vi "Get XY graph from TDMS file.vi"(8 "error in":errorcluster, 11 "TDMS file path":path) -> (0 "error out":errorcluster, 1 "graph":cluster{"X":dbl[], "Y":dbl[]}[](graph), 3 "TDMS file path out":path)   [LabVIEW 2025]
panel:
  out "Numeric":i32
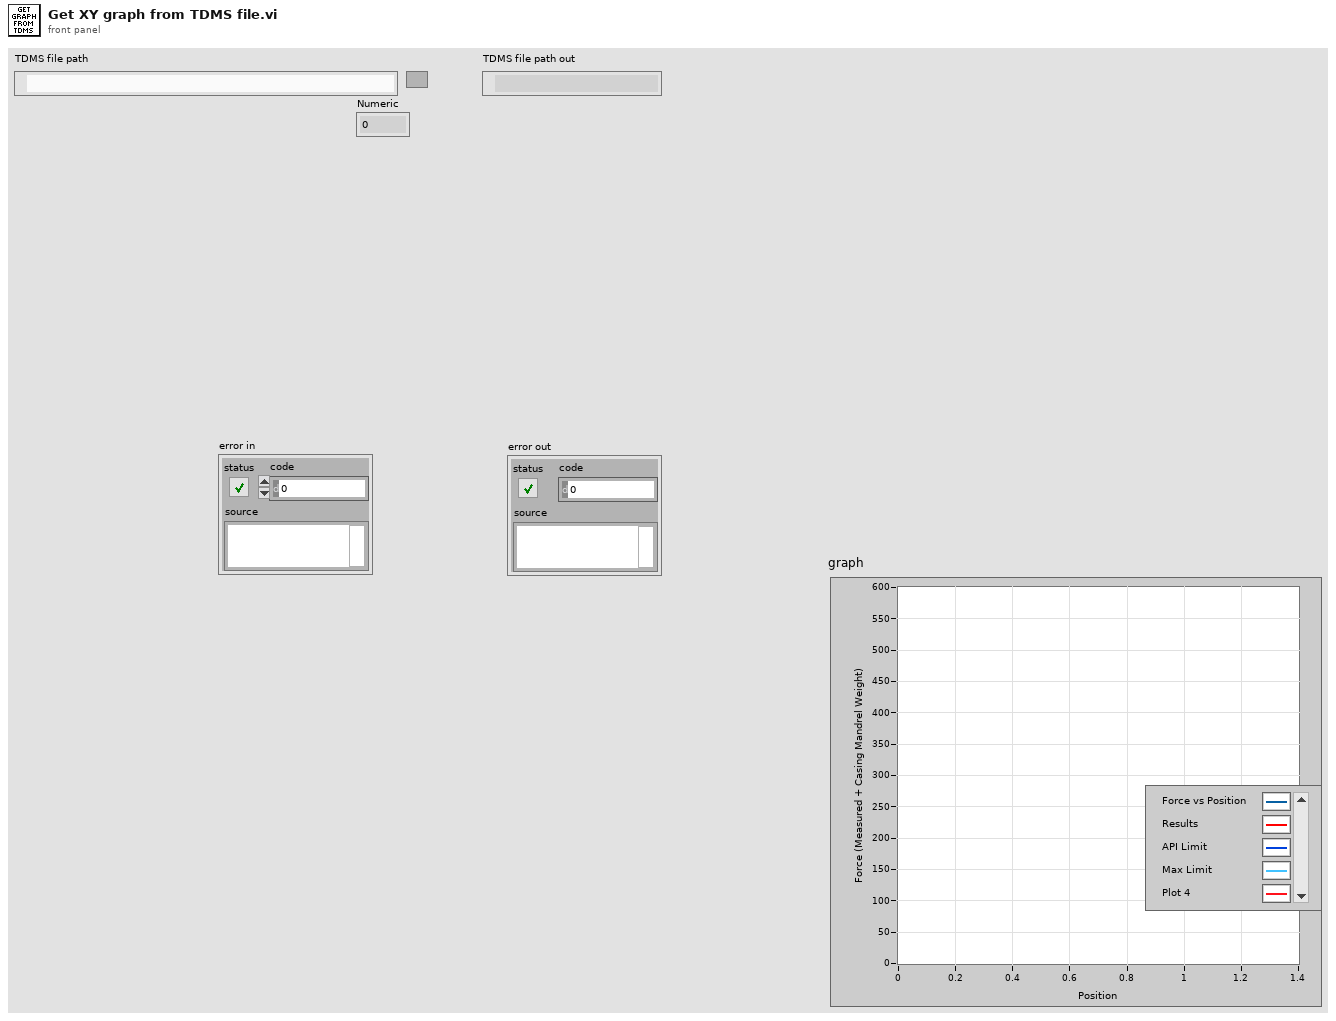
[diagram p1: front panel]
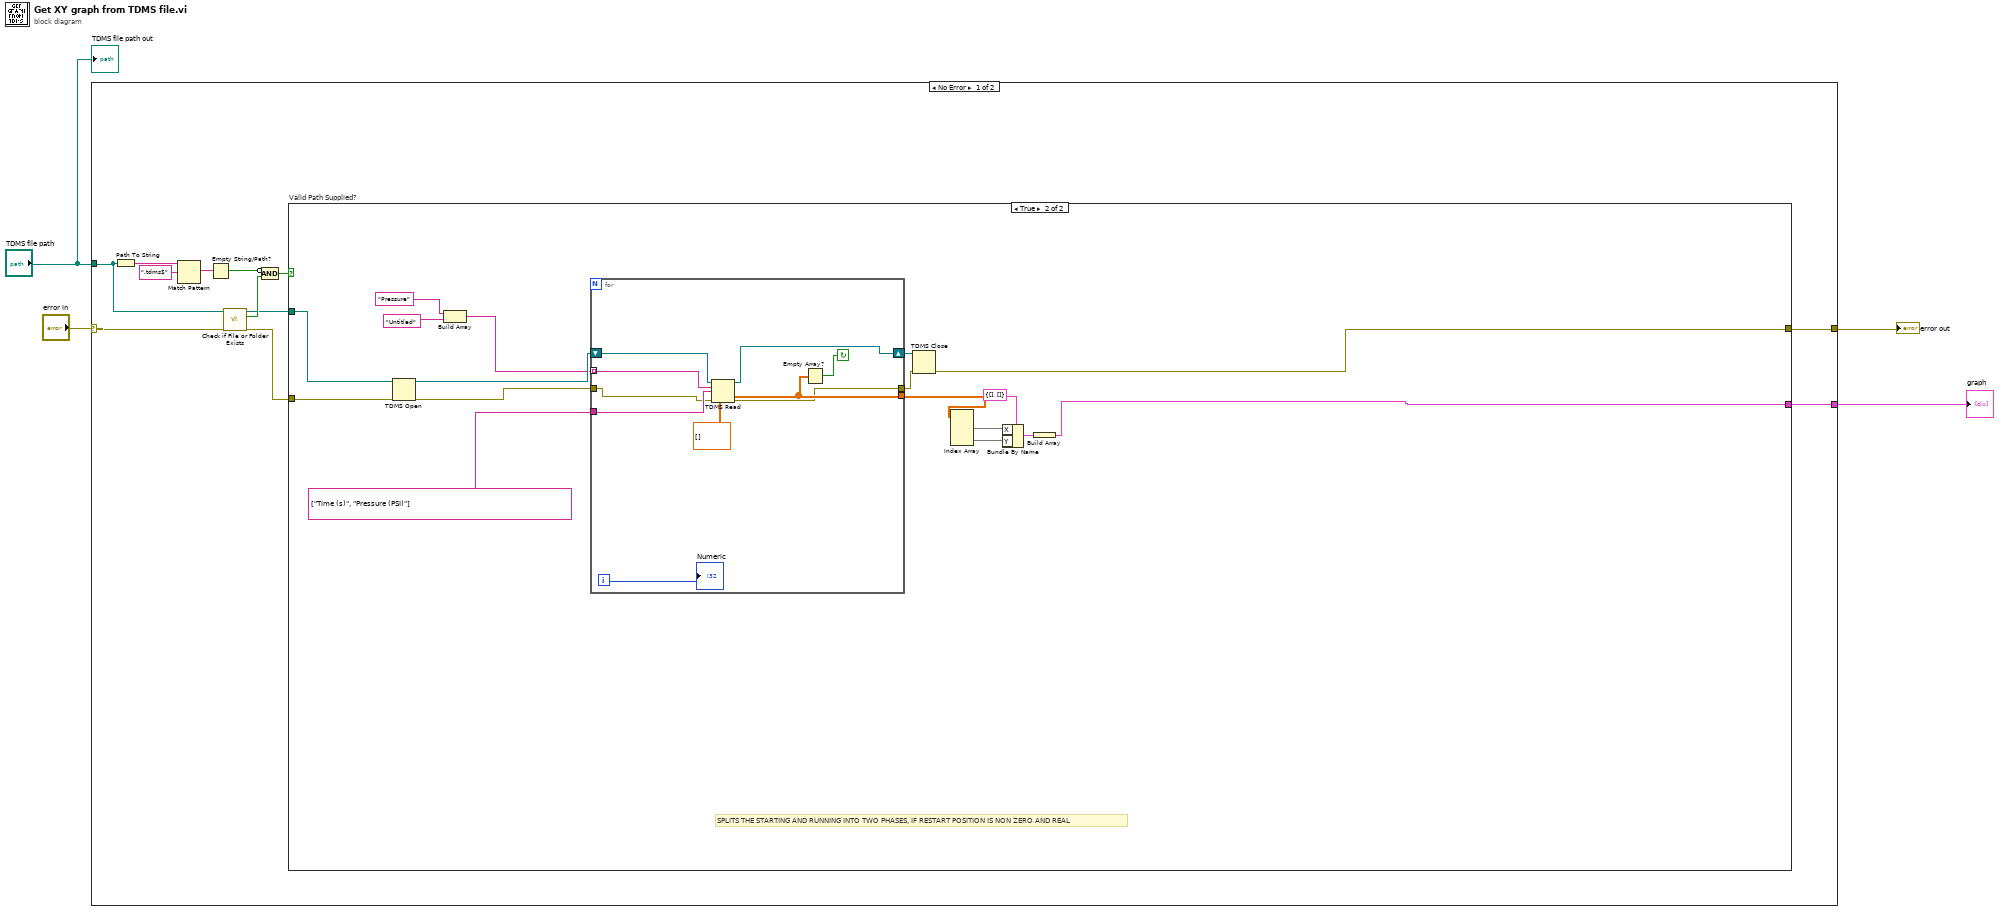
[diagram p0: block diagram]
diagram:
  n1 = case shown="No Error" "error in" {
    selector: "error in" -> [w5 w45]
    tunnel: "TDMS file path" -> [w14 _]
    tunnel: [w9 w45] -> w2
    tunnel: [w8 _] -> w1
    frame No Error {
      n2 = Path To String(path=w14) -> (string=w15:string)
      n3 = Match Pattern(string=w15, regular expression=".tdms$") -> (match substring=w13:string)  [unwired: 1 in, 3 out]
      n4 = Empty String/Path?(string/path=w13) -> (empty?=w12:bool)
      n5 = call <vilib>:"Check if File or Folder Exists.vi"("error in (no error)"=w5, "path"=w14) -> ("error out"=w6:errorcluster, "file or folder exists?"=w11:bool, "dup path"=w7:path)  [unwired: 7 in]
      n6 = Compound Arithmetic op=AND(invert w12, w11) -> (w10:bool)
      n7 = case "Valid Path Supplied?" shown="True" w10 {
        tunnel: [w17 w19] -> w9
        tunnel: [_ w25] -> w8
        tunnel: w7 -> [_ w32]
        tunnel: w6 -> [w17 w31]
        frame False {
          # "no need to notify the user, \nfile level properties vi should have already done that."
        }
        frame True {
          # "SPLITS THE STARTING AND RUNNING INTO TWO PHASES, IF RESTART POSITION IS NON ZERO AND REAL"
          n8 = TDMS Open(8:w31, 11:w32) -> (0:w34:errorcluster, 3:w33:refnum<k34>)  [unwired: 5 in]
          n9 = Build Array("Pressure" ("group name in"), "Untitled" ("group name in")) -> (w21:string[])
          n10 = for {
            tunnel: w21 -> [w43] mode=indexing
            tunnel: string[] ["Time (s)", "Pressure (PSI)"] ("channel name(s) in") -> [w40]
            tunnel: [w41] -> w24
            shift-right: [w37] -> w20
            shift-left: w33 -> [w44]
            tunnel: w34 -> [w35]
            tunnel: [w36] -> w18
            i -> [w38]
            stop <- w39 continue-if-true
            n11 = TDMS Read(0:w44, 5:w43, 7:w40, 11:w35, 12:dbl[][] [] ("Array")) -> (4:w37:refnum<k34>, 10:w41:dbl[][], 15:w36:errorcluster)  [unwired: 3 in, 3 out]
            n12 = Empty Array?(array=w41) -> (empty?=w39:bool)
            "Numeric" <- w38
          }
          n13 = TDMS Close(8:w18, 11:w20) -> (0:w19:errorcluster)  [unwired: 1 out]
          n14 = Index Array(array=w24) -> (element #1=w28:dbl[], element #2=w27:dbl[])  [unwired: 4 in]
          n15 = Bundle By Name(cluster=cluster{"X":dbl[], "Y":dbl[]} {"X"=[], "Y"=[]} ("Running Force Line"), "X"=w28, "Y"=w27) -> (w26:cluster{"X":dbl[], "Y":dbl[]})
          n16 = Build Array(w26) -> (w25:cluster{"X":dbl[], "Y":dbl[]}[])
        }
      }
    }
    frame Error {
    }
  }
  "error out" <- w2
  "graph" <- w1
  "TDMS file path out" <- "TDMS file path"
